vi "PolarizationSimulation.vi"() -> ()   [LabVIEW 2018]
uses:
  <vilib>/Utility/xml.llb/Read From XML File(string).vi
  <vilib>/Utility/xml.llb/Write to XML File(string).vi
  <vilib>/Analysis/NI_AALBase.lvlib
panel:
  out "NN Testing Error":dbl(graph)
  in  "Optimizer":enum16{"Adagrad", "Adadelta", "Adam"}(ring)
  in  "Loss Function":enum16{"MSE", "MAE"}(ring)
  in  "Parameters File Path":path
  out "NN Error":dbl
  in  "Training?":bool
  out "NN Output":dbl
  in  "Speed\nMultiplier":dbl=1.0
  out "Rho_-":cluster{dbl[], "Array 3":dbl[]}(graph)
  out "Rho_0":cluster{dbl[], "Array out":dbl[]}(graph)
  in  "AFP On":bool
  in  "AFP Efficiency":dbl=0.9 min=0.0 max=1.0 step=0.01
  in  "AFP Control":cluster{i32, i32}(slide)={200, 230} scale=0.0..500.0
  out "lower R-value AFP":dbl
  out "upper R-value AFP":dbl
  in  "STOP":bool
  in  "Microwave Power":dbl=1.0
  in  "Lower Fit\nParameter":dbl=-3.6
  in  "Upper Fit\nParameter":dbl=3.6
  in  "Std Dev Noise":dbl step=0.0001
  out "lower R-value":dbl
  out "upper R-value":dbl
  in  "RF Control":cluster{i32, i32}(slide)={200, 230} scale=0.0..500.0
  out "p":dbl format="%_4g"
  out "r":dbl
  in  "Saturation\nPolarization":dbl=0.8 min=0.0 max=0.99 step=0.01
  out "Reimann \nsum of Q":dbl format="%_4g"
  out "Corrected Data (Q)":cluster{dbl[], dbl[]}(graph)
  out "Rho_+":cluster{dbl[], "Array out":dbl[]}(graph)
  in  "Select Target Type":u16(ring)=2 items=["Test Case", "Deuteron"]
  in  "Reset":bool
  out "Total Polarization (P)":cluster{dbl, dbl}(graph)
  in  "Spin Manipulation\nPower Factor":dbl=0.005
  in  "Decay Spin\nManipulation":bool
  out "Reimann\nsum of P":dbl format="%_4g"
  out "Corrected Data (P)":cluster{dbl[], dbl[]}[](graph)
  out "Signal and Fit (P)":cluster{dbl[], "Best Polynomial Fit":dbl[]}[](graph)
  in  "Positive\nPolarization":bool
  in  "Microwave on":bool
  # "Neural Network"
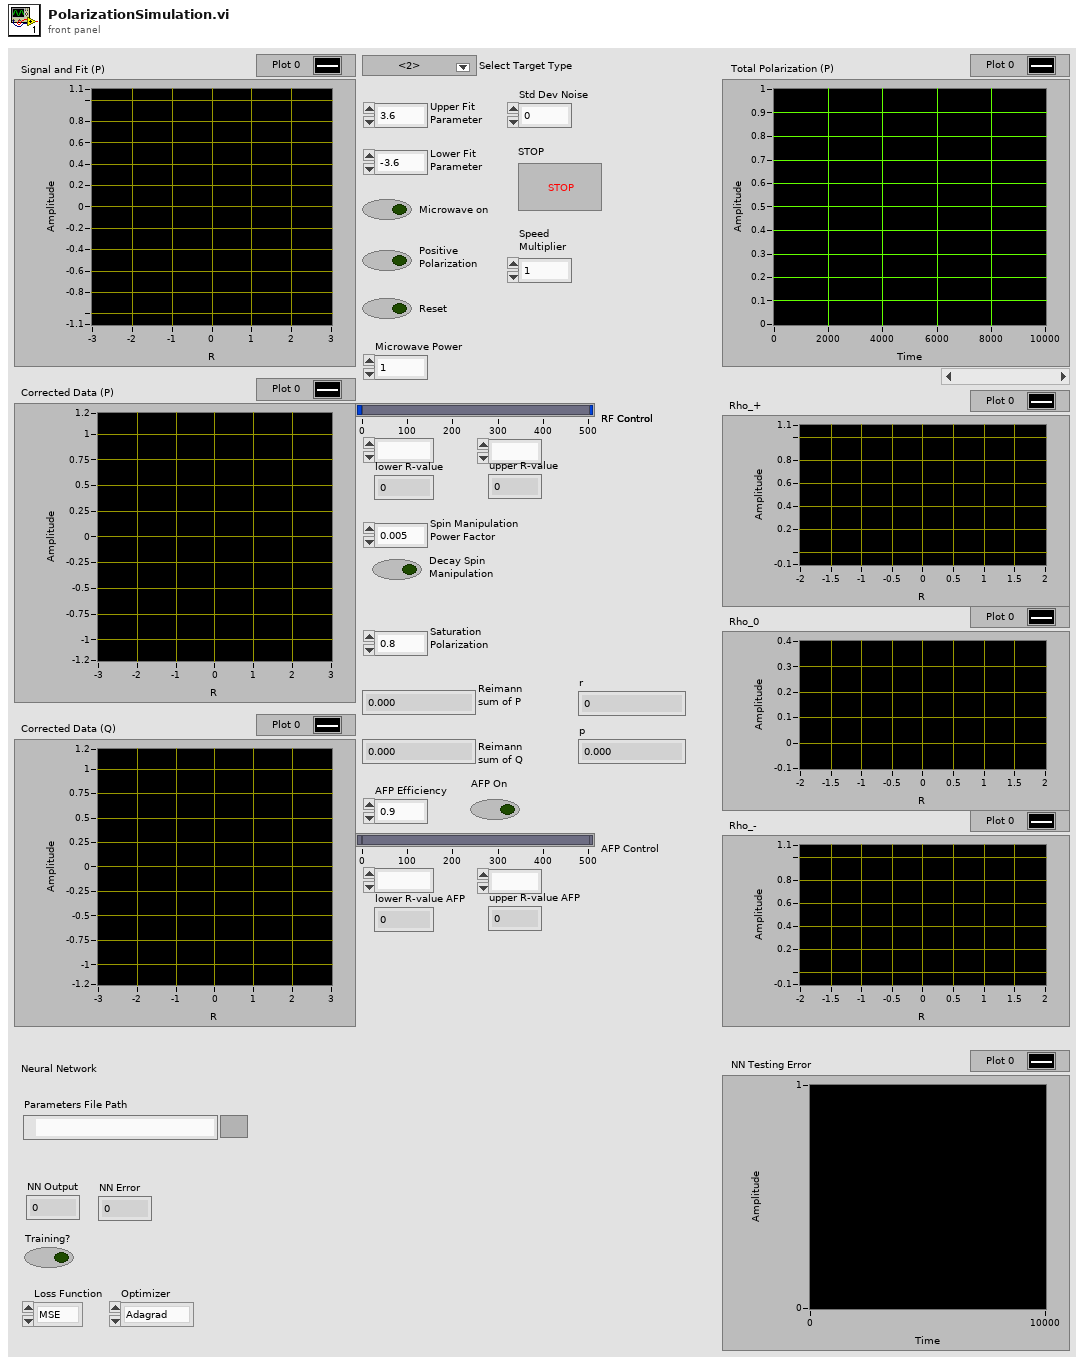
[diagram p1: front panel]
types:
  T1 = cluster{"Mw Moments":cluster{"3 ":dbl[], "2":dbl[][], "1":dbl[][]}, "Vw Moments":cluster{"3":dbl[], "2":dbl[][], "1":dbl[][]}, "Mb Moments":cluster{"1":dbl[], "2":dbl[], "3":dbl}, "Vb Moments":cluster{"3":dbl, "2":dbl[], "1":dbl[]}}
  T2 = cluster{cluster{dbl[][], dbl[]}, cluster{dbl[][], dbl[]}, cluster{dbl[], dbl}}
  T3 = cluster{cluster{"Updated Weights":dbl[][], "Updated Biases":dbl[]}, cluster{"Updated Weights":dbl[][], "Updated Biases":dbl[]}, cluster{"Updated Weights":dbl[], "Updated Biases":dbl}}
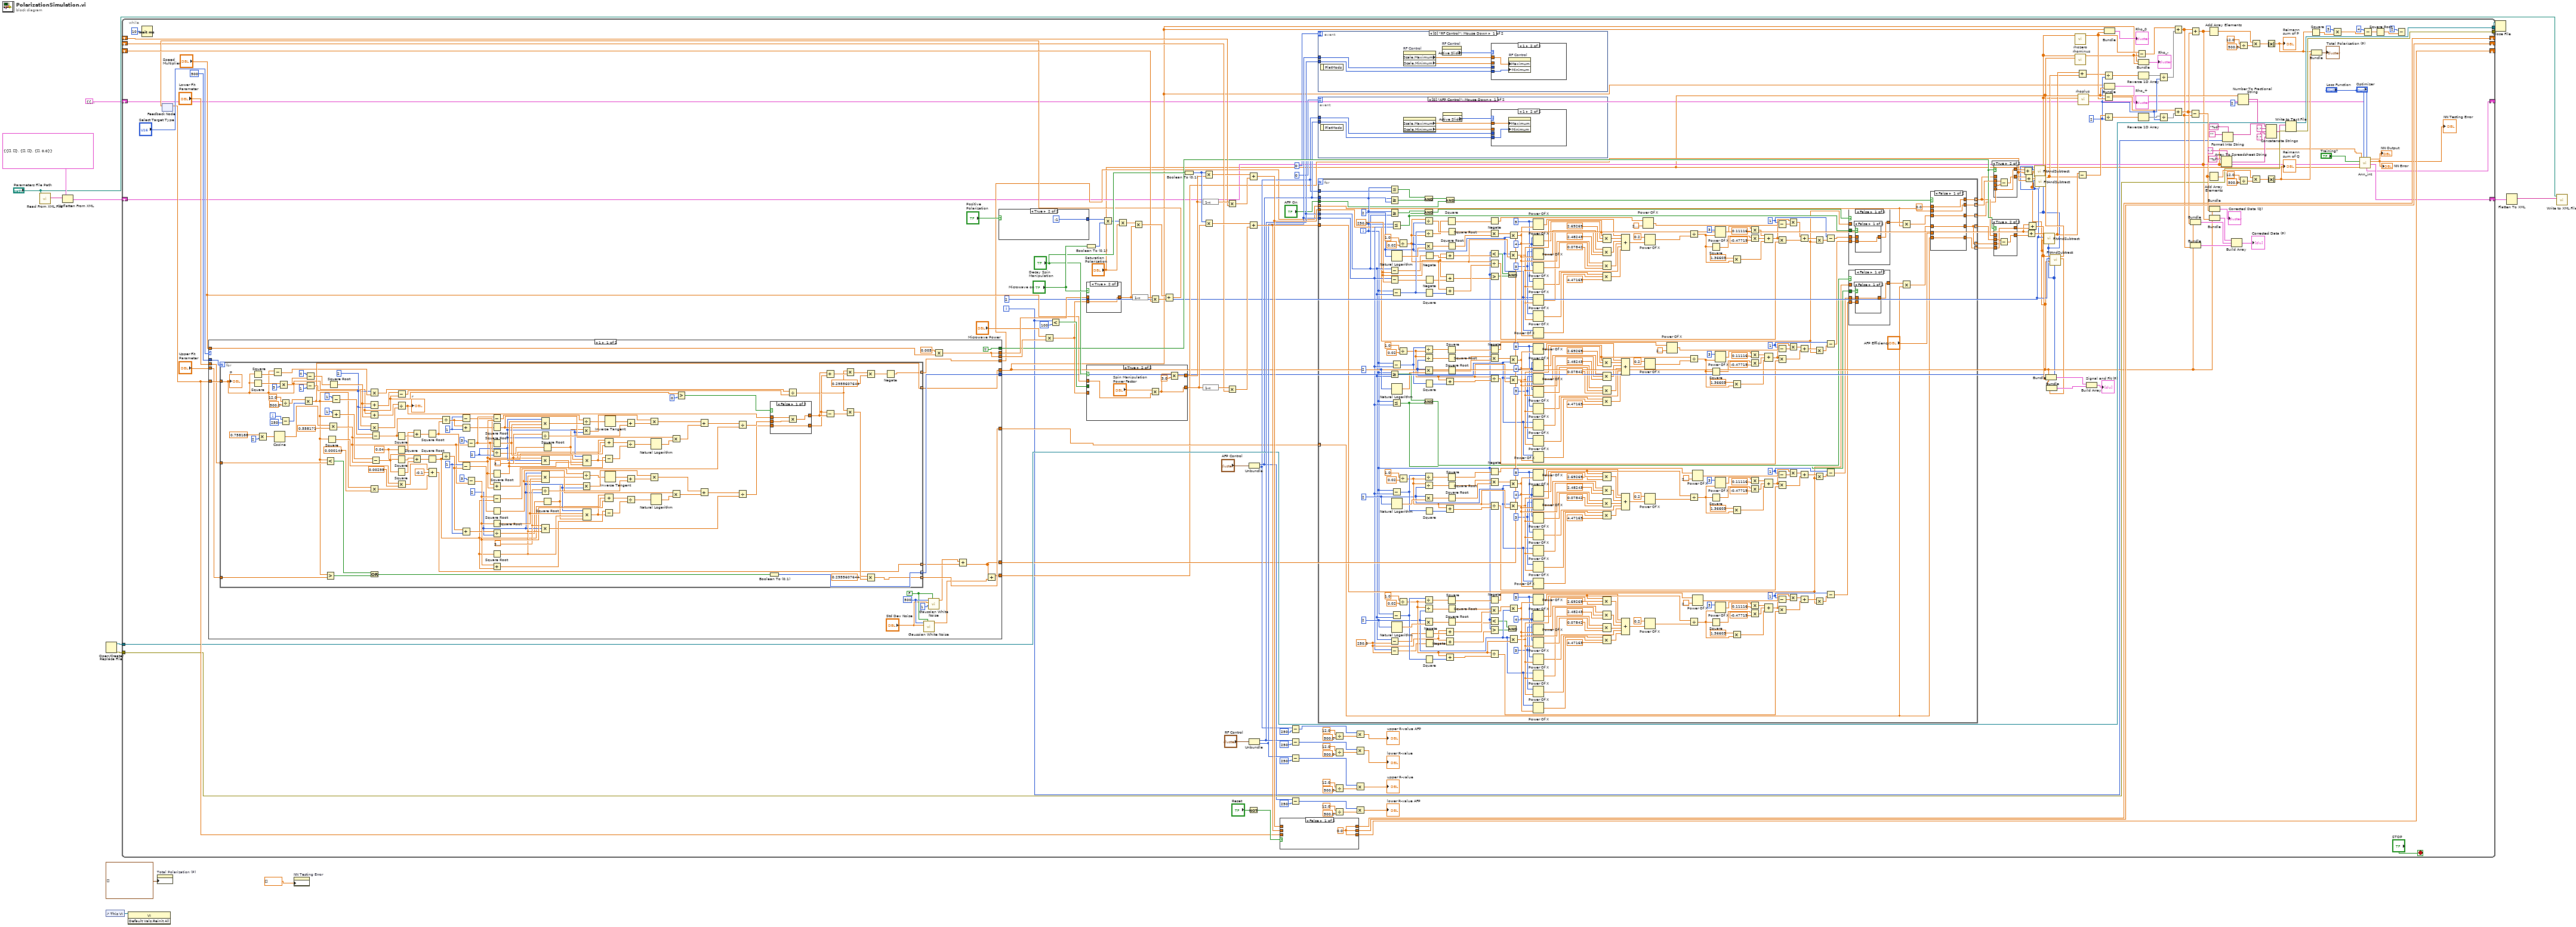
[diagram p0: block diagram]
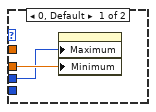
[diagram p2: hidden frame]
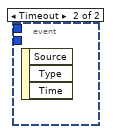
[diagram p3: hidden frame]
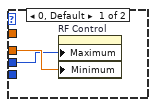
[diagram p4: hidden frame]
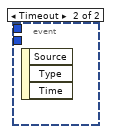
[diagram p5: hidden frame]
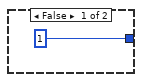
[diagram p6: hidden frame]
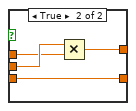
[diagram p7: hidden frame]
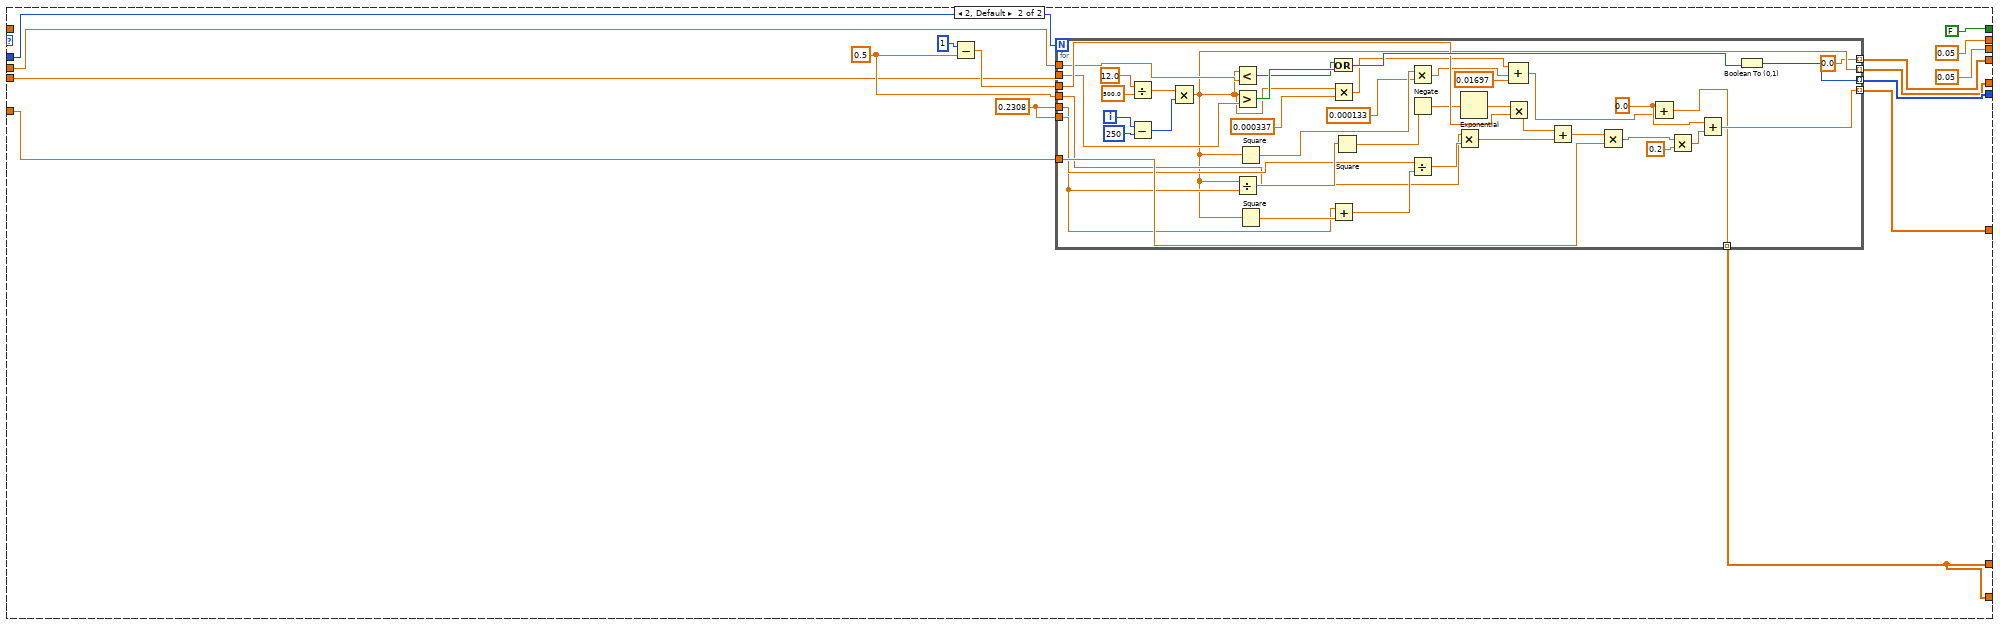
[diagram p8: hidden frame]
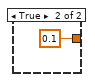
[diagram p10: hidden frame]
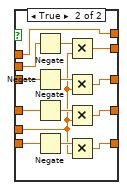
[diagram p15: hidden frame]
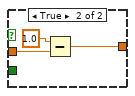
[diagram p17: hidden frame]
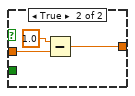
[diagram p19: hidden frame]
diagram:
  n1 = call-poly <vilib>:"Read From XML File.vi"("XML File Path"="Parameters File Path") -> ("XML Elements"=w8:string)  [unwired: 8 in, 2 out]
  n2 = Unflatten From XML(xml string=w8, type=T2 {{[], []}, {[], []}, {[], 0.0}}) -> (value=w6:T2)  [unwired: 1 in, 1 out]
  n3 = Open/Create/Replace File() -> (refnum out=w12:refnum<file>, error out=w11:errorcluster)  [unwired: 6 in, 1 out]
  n4 = control-ref of="This VI"() -> (w14:refnum<vi>)
  n5 = while {
    shift-right: [w181] -> _
    shift-left: _ -> [w188]
    shift-right: [w180] -> _
    shift-left: _ -> [w163]
    shift-right: [w158] -> _
    shift-left: _ -> [w157]
    tunnel: w12 -> [w90]
    tunnel: w11 -> [w89]
    tunnel: [w88] -> w10
    tunnel: [w87] -> w9
    shift-right: [w25] -> w5
    shift-left: w6 -> [w24]
    shift-right: [w17] -> _
    shift-left: T1 {"Mw Moments"={"3 "=[], "2"=[], "1"=[]}, "Vw Moments"={"3"=[], "2"=[], "1"=[]}, "Mb Moments"={"1"=[], "2"=[], "3"=0.0}, "Vb Moments"={"3"=0.0, "2"=[], "1"=[]}} -> [w18]
    i -> [w16]
    stop <- "STOP" stop-if-true
    w140 = 2
    w33 = 2
    n6 = Wait (ms)(milliseconds to wait=10) -> ()  [unwired: 1 out]
    n7 = feedback #1() -> (w167:dbl)  [unwired: 1 in]
    n8 = case shown="1" "Select Target Type" {
      tunnel: [w223 0.05 ("Growth Constant")] -> w172
      tunnel: [w223 0.05 ("Decay Constant")] -> w171
      tunnel: 500 -> [w232 w390]
      tunnel: w167 -> [w235 w389]
      tunnel: "Upper Fit\nParameter" -> [w233 w387]
      tunnel: "Lower Fit\nParameter" -> [w234 w388]
      tunnel: [w230 w385] -> w32
      tunnel: [w220 w384] -> w47
      tunnel: [w231 w386] -> w31
      tunnel: [TRUE FALSE] -> w151
      tunnel: [w221 w380] -> w46
      tunnel: "Speed\nMultiplier" -> [w222 _]
      tunnel: [w216 w379] -> w45
      tunnel: [w218 w379] -> w44
      frame 1 {
        w225 = FALSE
        w227 = 500
        n9 = for {
          N: w232 -> [_]
          tunnel: [w266] -> w230 mode=indexing
          tunnel: [w355] -> w231 mode=indexing
          tunnel: w233 -> [w354]
          tunnel: w234 -> [w353]
          tunnel: [w238] -> w220 mode=indexing
          tunnel: w235 -> [w239]
          tunnel: [w237] -> w221 mode=indexing
          tunnel: [w236] -> w219 mode=indexing
          i -> [w331]
          w253 = 2
          w292 = 1
          w296 = 3.141592653589793
          w290 = 2
          w275 = 0.04
          w328 = 1
          w333 = 3.141592653589793
          w326 = 2
          n10 = Square(x=w239) -> (x^2=w256:dbl)
          n11 = Square(x=w239) -> (x^2=w282:dbl)
          n12 = Multiply(x=0.758188, y=2) -> (x*y=w270:dbl)
          n13 = Subtract(x=w239, y=w256) -> (x-y=w255:dbl)
          n14 = Cosine(x=w270) -> (cos(x)=w273:dbl)
          n15 = Multiply(x=w282, y=3) -> (x*y=w281:dbl)
          n16 = Divide(x=12.0, y=500.0) -> (x/y=w369:dbl)
          n17 = Subtract(x=w331, y=250) -> (x-y=w368:i32)
          n18 = Multiply(x=w369, y=w368) -> (x*y=w266:dbl)
          n19 = Subtract(x=4, y=w281) -> (x-y=w279:dbl)
          n20 = Subtract(x=w239, y=1) -> (x-y=w277:dbl)
          n21 = Less?(x=w266, y=w353) -> (x < y?=w358:bool)
          n22 = Greater?(x=w266, y=w354) -> (0:w357:bool)
          n23 = Square(x=w266) -> (x^2=w268:dbl)
          n24 = Multiply(x=w273, y=0.558171) -> (x*y=w274:dbl)
          n25 = Square Root(x=w279) -> (sqrt(x)=w254:dbl)
          n26 = Subtract(x=1, y=w266) -> (x-y=w363:dbl)
          n27 = Add(x=1, y=w266) -> (x+y=w320:dbl)
          n28 = Multiply(x=w253, y=w255) -> (x*y=w251:dbl)
          n29 = Add(x=w254, y=w253) -> (x+y=w252:dbl)
          n30 = Add(x=w239, y=w254) -> (x+y=w278:dbl)
          n31 = Multiply(x=w277, y=w253) -> (x*y=w261:dbl)
          n32 = Multiply(x=w266, y=0.000144) -> (x*y=w263:dbl)
          n33 = Or(x=w358, y=w357) -> (x .or. y?=w356:bool)
          n34 = Subtract(x=w363, y=w274) -> (x-y=w359:dbl)
          n35 = Subtract(x=w320, y=w274) -> (x-y=w316:dbl)
          n36 = Square(x=w359) -> (x^2=w362:dbl)
          n37 = Square(x=w275) -> (x^2=w361:dbl)
          n38 = Square(x=w275) -> (x^2=w318:dbl)
          n39 = Square(x=w316) -> (x^2=w319:dbl)
          n40 = Subtract(x=w252, y=w239) -> (x-y=w250:dbl)
          n41 = Divide(x=w278, y=w261) -> (x/y=w257:dbl)
          "r" <- w257
          n42 = Multiply(x=w268, y=0.00295) -> (x*y=w267:dbl)
          n43 = Add(x=w361, y=w362) -> (x+y=w360:dbl)
          n44 = Add(x=w318, y=w319) -> (x+y=w317:dbl)
          n45 = Square Root(x=w360) -> (sqrt(x)=w323:dbl)
          n46 = Square Root(x=w317) -> (sqrt(x)=w287:dbl)
          n47 = Compound Arithmetic op=ADD(w267, -0.1, w263) -> (w236:dbl)
          n48 = Divide(x=w359, y=w323) -> (x/y=w329:dbl)
          n49 = Divide(x=w316, y=w287) -> (x/y=w293:dbl)
          n50 = Subtract(x=w328, y=w329) -> (x-y=w284:dbl)
          n51 = Add(x=w329, y=w328) -> (x+y=w327:dbl)
          n52 = Subtract(x=w292, y=w293) -> (x-y=w285:dbl)
          n53 = Add(x=w293, y=w292) -> (x+y=w291:dbl)
          n54 = Subtract(x=3, y=w274) -> (x-y=w339:dbl)
          n55 = Subtract(x=3, y=w274) -> (x-y=w302:dbl)
          n56 = Subtract(x=w339, y=w323) -> (x-y=w348:dbl)
          n57 = Square Root(x=w284) -> (sqrt(x)=w330:dbl)
          n58 = Square Root(x=w339) -> (sqrt(x)=w342:dbl)
          n59 = Divide(x=w327, y=w326) -> (x/y=w325:dbl)
          n60 = Square Root(x=w323) -> (sqrt(x)=w332:dbl)
          n61 = Add(x=w339, y=w323) -> (x+y=w338:dbl)
          n62 = Subtract(x=w302, y=w287) -> (x-y=w311:dbl)
          n63 = Square Root(x=w285) -> (sqrt(x)=w294:dbl)
          n64 = Square Root(x=w302) -> (sqrt(x)=w305:dbl)
          n65 = Divide(x=w291, y=w290) -> (x/y=w289:dbl)
          n66 = Square Root(x=w287) -> (sqrt(x)=w295:dbl)
          n67 = Add(x=w302, y=w287) -> (x+y=w301:dbl)
          n68 = Divide(x=w333, y=w326) -> (x/y=w350:dbl)
          n69 = Divide(x=w296, y=w290) -> (x/y=w313:dbl)
          n70 = Compound Arithmetic op=MULTIPLY(w326, w332, w342, w330) -> (w347:dbl)
          n71 = Compound Arithmetic op=MULTIPLY(w333, w326, w332) -> (w334:dbl)
          n72 = Compound Arithmetic op=MULTIPLY(w290, w295, w305, w294) -> (w310:dbl)
          n73 = Compound Arithmetic op=MULTIPLY(w296, w290, w295) -> (w297:dbl)
          n74 = Square Root(x=w325) -> (sqrt(x)=w324:dbl)
          n75 = Square Root(x=w289) -> (sqrt(x)=w288:dbl)
          n76 = Divide(x=w348, y=w347) -> (x/y=w346:dbl)
          n77 = Multiply(x=w324, y=w326) -> (x*y=w352:dbl)
          n78 = Divide(x=w311, y=w310) -> (x/y=w309:dbl)
          n79 = Multiply(x=w288, y=w290) -> (x*y=w315:dbl)
          n80 = Compound Arithmetic op=MULTIPLY(w326, w342, w332, w324) -> (w337:dbl)
          n81 = Compound Arithmetic op=MULTIPLY(w290, w305, w295, w288) -> (w300:dbl)
          n82 = Subtract(x=w338, y=w337) -> (x-y=w336:dbl)
          n83 = Subtract(x=w301, y=w300) -> (x-y=w299:dbl)
          n84 = Inverse Tangent(1:w346) -> (0:w351:dbl)
          n85 = Compound Arithmetic op=ADD(w337, w323, w339) -> (w341:dbl)
          n86 = Inverse Tangent(1:w309) -> (0:w314:dbl)
          n87 = Compound Arithmetic op=ADD(w300, w287, w302) -> (w304:dbl)
          n88 = Add(x=w351, y=w350) -> (x+y=w349:dbl)
          n89 = Divide(x=w341, y=w336) -> (x/y=w340:dbl)
          n90 = Add(x=w314, y=w313) -> (x+y=w312:dbl)
          n91 = Divide(x=w304, y=w299) -> (x/y=w303:dbl)
          n92 = Multiply(x=w352, y=w349) -> (x*y=w345:dbl)
          n93 = Multiply(x=w315, y=w312) -> (x*y=w308:dbl)
          n94 = Natural Logarithm(1:w340) -> (0:w343:dbl)
          n95 = Natural Logarithm(1:w303) -> (0:w306:dbl)
          n96 = Multiply(x=w330, y=w343) -> (x*y=w344:dbl)
          n97 = Multiply(x=w294, y=w306) -> (x*y=w307:dbl)
          n98 = Greater?(x=w239, y=0) -> (0:w241:bool)
          n99 = Add(x=w345, y=w344) -> (x+y=w335:dbl)
          n100 = Add(x=w308, y=w307) -> (x+y=w298:dbl)
          n101 = Divide(x=w335, y=w334) -> (x/y=w276:dbl)
          n102 = Divide(x=w298, y=w297) -> (x/y=w243:dbl)
          n103 = Boolean To (0,1)(Boolean=w356) -> (0, 1=w355:i16)
          n104 = case shown="False" w241 {
            tunnel: w276 -> [w373 w378]
            tunnel: [w371 w377] -> w259
            tunnel: w257 -> [w374 w376]
            tunnel: w243 -> [w372 w375]
            tunnel: [w372 w375] -> w242
            frame False {
              n105 = Multiply(x=w374, y=w373) -> (x*y=w371:dbl)
            }
            frame True {
              n106 = Multiply(x=w378, y=w376) -> (x*y=w377:dbl)
            }
          }
          n107 = Divide(x=w251, y=w250) -> (x/y=w249:dbl)
          n108 = Add(x=w259, y=w242) -> (x+y=w260:dbl)
          n109 = Subtract(x=w242, y=w259) -> (x-y=w286:dbl)
          n110 = Multiply(x=w249, y=w260) -> (x*y=w248:dbl)
          n111 = Multiply(x=w249, y=w286) -> (x*y=w247:dbl)
          n112 = Multiply(x=w248, y=0.2955607644) -> (x*y=w246:dbl)
          n113 = Multiply(x=w247, y=0.2955607644) -> (x*y=w238:dbl)
          n114 = Negate(x=w246) -> (-x=w237:dbl)
          "p" <- w239
        }
        n115 = call <vilib>:"Gaussian White Noise.vi"("initialize?"=w225, "standard deviation"="Std Dev Noise", "samples"=w227) -> ("Gaussian noise pattern"=w217:dbl[])  [unwired: 7 in, 1 out]
        n116 = call <vilib>:"Gaussian White Noise.vi"("initialize?"=w225, "seed"=1, "standard deviation"="Std Dev Noise", "samples"=w227) -> ("Gaussian noise pattern"=w215:dbl[])  [unwired: 6 in, 1 out]
        n117 = Multiply(x=0.005, y=w222) -> (x*y=w223:dbl)
        n118 = Add(x=w215, y=w219) -> (x+y=w216:dbl[])
        n119 = Add(x=w216, y=w217) -> (x+y=w218:dbl[])
      }
      frame 2, Default {
        w391 = 0.2308
        w392 = 0.5
        n120 = Subtract(x=1, y=w392) -> (x-y=w394:dbl)
        n121 = for {
          N: w390 -> [_]
          tunnel: w389 -> [w434]
          tunnel: [w400] -> w385 mode=indexing
          tunnel: [w418] -> w384 mode=indexing
          tunnel: [w432] -> w386 mode=indexing
          tunnel: w394 -> [w428]
          tunnel: w391 -> [w426]
          tunnel: w391 -> [w407]
          tunnel: w392 -> [w420]
          tunnel: w387 -> [w415]
          tunnel: w388 -> [w414]
          tunnel: [0.0] -> w380 mode=indexing
          tunnel: [w395] -> w379 mode=indexing
          i -> [w408]
          w419 = 0.0
          n122 = Divide(x=12.0, y=500.0) -> (x/y=w409:dbl)
          n123 = Subtract(x=w408, y=250) -> (x-y=w413:i32)
          n124 = Multiply(x=w409, y=w413) -> (x*y=w400:dbl)
          n125 = Less?(x=w400, y=w414) -> (x < y?=w429:bool)
          n126 = Greater?(x=w400, y=w415) -> (0:w430:bool)
          n127 = Divide(x=w400, y=w407) -> (x/y=w435:dbl)
          n128 = Square(x=w400) -> (x^2=w403:dbl)
          n129 = Square(x=w400) -> (x^2=w425:dbl)
          n130 = Or(x=w429, y=w430) -> (x .or. y?=w431:bool)
          n131 = Multiply(x=w400, y=0.000337) -> (x*y=w402:dbl)
          n132 = Add(x=w407, y=w425) -> (x+y=w427:dbl)
          n133 = Square(x=w435) -> (x^2=w436:dbl)
          n134 = Multiply(x=w403, y=0.000133) -> (x*y=w401:dbl)
          n135 = Negate(x=w436) -> (-x=w417:dbl)
          n136 = Divide(x=w426, y=w427) -> (x/y=w422:dbl)
          n137 = Multiply(x=w420, y=w422) -> (x*y=w421:dbl)
          n138 = Exponential(1:w417) -> (0:w416:dbl)
          n139 = Multiply(x=w416, y=w428) -> (x*y=w424:dbl)
          n140 = Compound Arithmetic op=ADD(w402, w401, 0.01697) -> (w404:dbl)
          n141 = Add(x=w424, y=w421) -> (x+y=w423:dbl)
          n142 = Multiply(x=w423, y=w434) -> (x*y=w433:dbl)
          n143 = Add(x=w419, y=w404) -> (x+y=w395:dbl)
          n144 = Multiply(x=w433, y=0.2) -> (x*y=w406:dbl)
          n145 = Add(x=w419, y=w406) -> (x+y=w418:dbl)
          n146 = Boolean To (0,1)(Boolean=w431) -> (0, 1=w432:i16)
        }
      }
    }
    n147 = case shown="True" "Positive\nPolarization" {
      tunnel: [1 -1] -> w125
      frame False {
      }
      frame True {
      }
    }
    n148 = Multiply(x="Microwave Power", y=w172) -> (x*y=w93:dbl)
    n149 = Less?(x=w16, y=100) -> (x < y?=w183:bool)
    n150 = Boolean To (0,1)(Boolean="Microwave on") -> (0, 1=w190:i16)
    n151 = case shown="True" "Microwave on" {
      tunnel: [w447 w448] -> w175
      tunnel: w93 -> [_ w448]
      tunnel: w171 -> [w447 _]
      frame False {
      }
      frame True {
      }
    }
    n152 = case shown="True" "Decay Spin\nManipulation" {
      tunnel: [w437 w443] -> w184
      tunnel: w93 -> [w439 _]
      tunnel: w183 -> [w438 _]
      tunnel: [w437 w444] -> w165
      tunnel: "Speed\nMultiplier" -> [_ w442]
      frame False {
        n153 = case shown="False" w438 {
          tunnel: [w440 0.1] -> w437
          tunnel: w439 -> [w440 _]
          frame False {
          }
          frame True {
          }
        }
      }
      frame True {
        n154 = Multiply(x="Spin Manipulation\nPower Factor", y=w442) -> (x*y=w443:dbl)
        n155 = Multiply(x=w443, y=3.0) -> (x*y=w444:dbl)
      }
    }
    n156 = Multiply(x=w125, y=w190) -> (x*y=w126:i32)
    n157 = Multiply(x=w126, y="Saturation\nPolarization") -> (x*y=w133:dbl)
    n158 = expression code="1-x"(w175) -> (w191:dbl)
    n159 = Multiply(x=w133, y=w175) -> (x*y=w192:dbl)
    n160 = Multiply(x=w191, y=w188) -> (x*y=w193:dbl)
    n161 = Add(x=w192, y=w193) -> (x+y=w170:dbl)
    n162 = feedback-in #1(w170) -> ()
    n163 = Boolean To (0,1)(Boolean="Decay Spin\nManipulation") -> (0, 1=w166:i16)
    n164 = expression code="1-x"(w165) -> (w164:dbl)
    n165 = expression code="1-x"(w184) -> (w185:dbl)
    n166 = Multiply(x=w166, y=w165) -> (x*y=w161:dbl)
    n167 = Multiply(x=w166, y=w184) -> (x*y=w186:dbl)
    n168 = Multiply(x=w164, y=w157) -> (x*y=w162:dbl)
    n169 = Multiply(x=w185, y=w163) -> (x*y=w187:dbl)
    n170 = Add(x=w161, y=w162) -> (x+y=w159:dbl)
    n171 = Add(x=w186, y=w187) -> (x+y=w179:dbl)
    n172 = Not(x="Reset") -> (.not. x?=w178:bool)
    n173 = Unbundle("AFP Control") -> (w57:i32, w56:i32)
    n174 = Unbundle("RF Control") -> (w96:i32, w95:i32)
    n175 = case shown="False" w178 {
      tunnel: [w461 w464] -> w181
      tunnel: w167 -> [_ w464]
      tunnel: [w461 w463] -> w180
      tunnel: w179 -> [_ w463]
      tunnel: w159 -> [_ w462]
      tunnel: [w461 w462] -> w158
      frame False {
        w461 = 0.0
      }
      frame True {
      }
    }
    n176 = Subtract(x=w56, y=250) -> (x-y=w63:i32)
    n177 = Subtract(x=w96, y=250) -> (x-y=w102:i32)
    n178 = Subtract(x=w95, y=250) -> (x-y=w105:i32)
    n179 = Subtract(x=w57, y=250) -> (x-y=w60:i32)
    n180 = event shown="[0] \"RF Control\": Mouse Down" {
      selector: _ -> [_ _]
      dyn-events: _ -> [_ _]
      timeout: 0 -> [_ _]
      tunnel: w96 -> [w205 _]
      tunnel: w95 -> [w204 _]
      event "RF Control": Mouse Down {
        n181 = event-data() -> ()  [unwired: 1 in, 1 out]
        n182 = property on="RF Control" class="Slide (strict)"() -> ("Scale.Maximum"=w206:dbl, "Scale.Minimum"=w207:dbl)  [unwired: 2 in, 2 out]
        n183 = property on="RF Control" class="Slide (strict)"() -> ("Active Slider"=w208:i32)  [unwired: 2 in, 2 out]
        n184 = case shown="1" w208 {
          tunnel: w207 -> [w210 _]
          tunnel: w204 -> [w209 _]
          tunnel: w206 -> [_ w212]
          tunnel: w205 -> [_ w211]
          frame 0, Default {
            n185 = property on="RF Control" class="Slide (strict)"("Maximum"=w209, "Minimum"=w210) -> ()  [unwired: 2 in, 2 out]
          }
          frame 1 {
            n186 = property on="RF Control" class="Slide (strict)"("Maximum"=w212, "Minimum"=w211) -> ()  [unwired: 2 in, 2 out]
          }
        }
      }
      event Timeout {
        n187 = event-data() -> ()  [unwired: 1 in, 3 out]
      }
    }
    n188 = event shown="[0] \"AFP Control\": Mouse Down" {
      selector: _ -> [_ _]
      dyn-events: _ -> [_ _]
      timeout: 0 -> [_ _]
      tunnel: w57 -> [w196 _]
      tunnel: w56 -> [w195 _]
      event "AFP Control": Mouse Down {
        n189 = event-data() -> ()  [unwired: 1 in, 1 out]
        n190 = property on="AFP Control" class="Slide (strict)"() -> ("Scale.Maximum"=w197:dbl, "Scale.Minimum"=w198:dbl)  [unwired: 2 in, 2 out]
        n191 = property on="AFP Control" class="Slide (strict)"() -> ("Active Slider"=w199:i32)  [unwired: 2 in, 2 out]
        n192 = case shown="1" w199 {
          tunnel: w198 -> [w201 _]
          tunnel: w195 -> [w200 _]
          tunnel: w197 -> [_ w203]
          tunnel: w196 -> [_ w202]
          frame 0, Default {
            n193 = property on="AFP Control" class="Slide (strict)"("Maximum"=w200, "Minimum"=w201) -> ()  [unwired: 2 in, 2 out]
          }
          frame 1 {
            n194 = property on="AFP Control" class="Slide (strict)"("Maximum"=w203, "Minimum"=w202) -> ()  [unwired: 2 in, 2 out]
          }
        }
      }
      event Timeout {
        n195 = event-data() -> ()  [unwired: 1 in, 3 out]
      }
    }
    n196 = for {
      tunnel: w47 -> [w477] mode=indexing
      tunnel: w179 -> [w629]
      tunnel: w95 -> [w487]
      tunnel: w96 -> [w486]
      tunnel: [w473] -> w169 mode=indexing
      tunnel: [w474] -> w160 mode=indexing
      tunnel: [w474] -> w168 mode=indexing
      tunnel: w46 -> [w466] mode=indexing
      tunnel: w159 -> [w485]
      tunnel: [w465] -> w155 mode=indexing
      tunnel: [w472] -> w145 mode=indexing
      tunnel: w57 -> [w481]
      tunnel: w56 -> [w480]
      tunnel: "AFP On" -> [w469]
      tunnel: [w468] -> w54 mode=indexing
      i -> [w479]
      w489 = 250.0
      w528 = 5
      w526 = 4
      w525 = 3
      w506 = 1
      w507 = 2
      w589 = 5
      w587 = 4
      w586 = 3
      w566 = 1
      w567 = 2
      w623 = 250.0
      w664 = 5
      w662 = 4
      w661 = 3
      w642 = 1
      w643 = 2
      w725 = 5
      w723 = 4
      w722 = 3
      w702 = 1
      w703 = 2
      n197 = Less Or Equal?(x=w479, y=w480) -> (x <= y?=w482:bool)
      n198 = Greater Or Equal?(x=w479, y=w481) -> (x >= y?=w483:bool)
      n199 = Greater Or Equal?(x=w479, y=w486) -> (x >= y?=w562:bool)
      n200 = Subtract(x=w486, y=w489) -> (x-y=w493:dbl)
      n201 = Subtract(x=w487, y=w489) -> (x-y=w494:dbl)
      n202 = Greater Or Equal?(x=w479, y=w486) -> (x >= y?=w698:bool)
      n203 = Subtract(x=w486, y=w623) -> (x-y=w627:dbl)
      n204 = Subtract(x=w487, y=w623) -> (x-y=w628:dbl)
      n205 = Less Or Equal?(x=w479, y=w487) -> (x <= y?=w499:bool)
      n206 = Natural Logarithm(1:w567) -> (0:w602:dbl)
      n207 = Subtract(x=w479, y=w486) -> (x-y=w575:i32)
      n208 = Subtract(x=w479, y=w487) -> (x-y=w514:i32)
      n209 = Natural Logarithm(1:w507) -> (0:w541:dbl)
      n210 = Less Or Equal?(x=w479, y=w487) -> (x <= y?=w634:bool)
      n211 = Subtract(x=w479, y=w487) -> (x-y=w650:i32)
      n212 = Natural Logarithm(1:w643) -> (0:w677:dbl)
      n213 = Subtract(x=w479, y=w486) -> (x-y=w711:i32)
      n214 = Natural Logarithm(1:w703) -> (0:w738:dbl)
      n215 = Divide(x=1.0, y=0.02) -> (x/y=w571:dbl)
      n216 = Divide(x=1.0, y=0.02) -> (x/y=w511:dbl)
      n217 = Divide(x=1.0, y=0.02) -> (x/y=w647:dbl)
      n218 = Divide(x=1.0, y=0.02) -> (x/y=w707:dbl)
      n219 = And(x=w482, y=w483) -> (x .and. y?=w471:bool)
      n220 = And(x=w562, y=w499) -> (x .and. y?=w500:bool)
      n221 = Divide(x=w571, y=w567) -> (x/y=w600:dbl)
      n222 = Divide(x=w575, y=w571) -> (x/y=w579:dbl)
      n223 = Multiply(x=w567, y=w602) -> (x*y=w603:dbl)
      n224 = Divide(x=w514, y=w511) -> (x/y=w518:dbl)
      n225 = Divide(x=w511, y=w507) -> (x/y=w539:dbl)
      n226 = Multiply(x=w507, y=w541) -> (x*y=w542:dbl)
      n227 = And(x=w698, y=w634) -> (x .and. y?=w636:bool)
      n228 = Divide(x=w650, y=w647) -> (x/y=w654:dbl)
      n229 = Divide(x=w647, y=w643) -> (x/y=w675:dbl)
      n230 = Multiply(x=w643, y=w677) -> (x*y=w678:dbl)
      n231 = Divide(x=w711, y=w707) -> (x/y=w715:dbl)
      n232 = Divide(x=w707, y=w703) -> (x/y=w736:dbl)
      n233 = Multiply(x=w703, y=w738) -> (x*y=w739:dbl)
      n234 = Square(x=w575) -> (x^2=w576:i32)
      n235 = Square(x=w514) -> (x^2=w515:i32)
      n236 = Square(x=w650) -> (x^2=w651:i32)
      n237 = Square(x=w711) -> (x^2=w712:i32)
      n238 = Negate(x=w493) -> (-x=w492:dbl)
      n239 = Negate(x=w494) -> (-x=w490:dbl)
      n240 = Negate(x=w627) -> (-x=w626:dbl)
      n241 = Negate(x=w628) -> (-x=w624:dbl)
      n242 = Add(x=w489, y=w492) -> (x+y=w491:dbl)
      n243 = Add(x=w489, y=w490) -> (x+y=w488:dbl)
      n244 = Add(x=w571, y=w576) -> (x+y=w577:dbl)
      n245 = Add(x=w511, y=w515) -> (x+y=w516:dbl)
      n246 = Add(x=w647, y=w651) -> (x+y=w652:dbl)
      n247 = Add(x=w623, y=w626) -> (x+y=w625:dbl)
      n248 = Add(x=w623, y=w624) -> (x+y=w622:dbl)
      n249 = Add(x=w707, y=w712) -> (x+y=w713:dbl)
      n250 = And(x=w471, y=w469) -> (x .and. y?=w470:bool)
      n251 = Square(x=w579) -> (x^2=w581:dbl)
      n252 = Square(x=w518) -> (x^2=w520:dbl)
      n253 = Square(x=w654) -> (x^2=w656:dbl)
      n254 = Square(x=w715) -> (x^2=w717:dbl)
      n255 = Square Root(x=w600) -> (sqrt(x)=w601:dbl)
      n256 = Square Root(x=w603) -> (sqrt(x)=w604:dbl)
      n257 = Square Root(x=w539) -> (sqrt(x)=w540:dbl)
      n258 = Square Root(x=w542) -> (sqrt(x)=w543:dbl)
      n259 = Square Root(x=w675) -> (sqrt(x)=w676:dbl)
      n260 = Square Root(x=w678) -> (sqrt(x)=w679:dbl)
      n261 = Square Root(x=w736) -> (sqrt(x)=w737:dbl)
      n262 = Square Root(x=w739) -> (sqrt(x)=w740:dbl)
      n263 = Negate(x=w581) -> (-x=w580:dbl)
      n264 = Multiply(x=w601, y=w604) -> (x*y=w595:dbl)
      n265 = Less?(x=w479, y=w491) -> (x < y?=w496:bool)
      n266 = Divide(x=w571, y=w577) -> (x/y=w574:dbl)
      n267 = Greater?(x=w479, y=w488) -> (0:w495:bool)
      n268 = Negate(x=w520) -> (-x=w519:dbl)
      n269 = Multiply(x=w540, y=w543) -> (x*y=w534:dbl)
      n270 = Divide(x=w511, y=w516) -> (x/y=w501:dbl)
      n271 = Negate(x=w656) -> (-x=w655:dbl)
      n272 = Multiply(x=w676, y=w679) -> (x*y=w670:dbl)
      n273 = Divide(x=w647, y=w652) -> (x/y=w637:dbl)
      n274 = Negate(x=w717) -> (-x=w716:dbl)
      n275 = Multiply(x=w737, y=w740) -> (x*y=w731:dbl)
      n276 = Less?(x=w479, y=w625) -> (x < y?=w631:bool)
      n277 = Greater?(x=w479, y=w622) -> (0:w630:bool)
      n278 = Divide(x=w707, y=w713) -> (x/y=w710:dbl)
      n279 = And(x=w496, y=w495) -> ()  [unwired: 1 out]
      n280 = And(x=w631, y=w630) -> ()  [unwired: 1 out]
      n281 = Multiply(x=w595, y=w567) -> (x*y=w619:dbl)
      n282 = Multiply(x=w567, y=w571) -> (x*y=w613:dbl)
      n283 = Multiply(x=w534, y=w507) -> (x*y=w558:dbl)
      n284 = Multiply(x=w507, y=w511) -> (x*y=w552:dbl)
      n285 = Multiply(x=w670, y=w643) -> (x*y=w694:dbl)
      n286 = Multiply(x=w643, y=w647) -> (x*y=w688:dbl)
      n287 = Multiply(x=w731, y=w703) -> (x*y=w755:dbl)
      n288 = Multiply(x=w703, y=w707) -> (x*y=w749:dbl)
      n289 = Power Of X(1:w619, 2:w589) -> (0:w606:dbl)
      n290 = Power Of X(1:w619, 2:w587) -> (0:w612:dbl)
      n291 = Power Of X(1:w619, 2:w586) -> (0:w614:dbl)
      n292 = Power Of X(1:w613, 2:w587) -> (0:w618:dbl)
      n293 = Power Of X(1:w613, 2:w589) -> (0:w607:dbl)
      n294 = Power Of X(1:w613, 2:w567) -> (0:w615:dbl)
      n295 = Power Of X(1:w613, 2:w586) -> (0:w616:dbl)
      n296 = Power Of X(1:w619, 2:w567) -> (0:w617:dbl)
      n297 = Power Of X(1:w558, 2:w528) -> (0:w545:dbl)
      n298 = Power Of X(1:w558, 2:w526) -> (0:w551:dbl)
      n299 = Power Of X(1:w558, 2:w525) -> (0:w553:dbl)
      n300 = Power Of X(1:w552, 2:w526) -> (0:w557:dbl)
      n301 = Power Of X(1:w552, 2:w528) -> (0:w546:dbl)
      n302 = Power Of X(1:w552, 2:w507) -> (0:w554:dbl)
      n303 = Power Of X(1:w552, 2:w525) -> (0:w555:dbl)
      n304 = Power Of X(1:w558, 2:w507) -> (0:w556:dbl)
      n305 = Power Of X(1:w694, 2:w664) -> (0:w681:dbl)
      n306 = Power Of X(1:w694, 2:w662) -> (0:w687:dbl)
      n307 = Power Of X(1:w694, 2:w661) -> (0:w689:dbl)
      n308 = Power Of X(1:w688, 2:w662) -> (0:w693:dbl)
      n309 = Power Of X(1:w688, 2:w664) -> (0:w682:dbl)
      n310 = Power Of X(1:w688, 2:w643) -> (0:w690:dbl)
      n311 = Power Of X(1:w688, 2:w661) -> (0:w691:dbl)
      n312 = Power Of X(1:w694, 2:w643) -> (0:w692:dbl)
      n313 = Power Of X(1:w755, 2:w725) -> (0:w742:dbl)
      n314 = Power Of X(1:w755, 2:w723) -> (0:w748:dbl)
      n315 = Power Of X(1:w755, 2:w722) -> (0:w750:dbl)
      n316 = Power Of X(1:w749, 2:w723) -> (0:w754:dbl)
      n317 = Power Of X(1:w749, 2:w725) -> (0:w743:dbl)
      n318 = Power Of X(1:w749, 2:w703) -> (0:w751:dbl)
      n319 = Power Of X(1:w749, 2:w722) -> (0:w752:dbl)
      n320 = Power Of X(1:w755, 2:w703) -> (0:w753:dbl)
      n321 = Compound Arithmetic op=MULTIPLY(w613, w612, 2.69269) -> (w608:dbl)
      n322 = Compound Arithmetic op=MULTIPLY(w614, w615, 2.48243) -> (w610:dbl)
      n323 = Compound Arithmetic op=MULTIPLY(w619, w618, 0.07842) -> (w609:dbl)
      n324 = Compound Arithmetic op=MULTIPLY(w616, w617, 4.47163) -> (w611:dbl)
      n325 = Compound Arithmetic op=MULTIPLY(w552, w551, 2.69269) -> (w547:dbl)
      n326 = Compound Arithmetic op=MULTIPLY(w553, w554, 2.48243) -> (w549:dbl)
      n327 = Compound Arithmetic op=MULTIPLY(w558, w557, 0.07842) -> (w548:dbl)
      n328 = Compound Arithmetic op=MULTIPLY(w555, w556, 4.47163) -> (w550:dbl)
      n329 = Compound Arithmetic op=MULTIPLY(w688, w687, 2.69269) -> (w683:dbl)
      n330 = Compound Arithmetic op=MULTIPLY(w689, w690, 2.48243) -> (w685:dbl)
      n331 = Compound Arithmetic op=MULTIPLY(w694, w693, 0.07842) -> (w684:dbl)
      n332 = Compound Arithmetic op=MULTIPLY(w691, w692, 4.47163) -> (w686:dbl)
      n333 = Compound Arithmetic op=MULTIPLY(w749, w748, 2.69269) -> (w744:dbl)
      n334 = Compound Arithmetic op=MULTIPLY(w750, w751, 2.48243) -> (w746:dbl)
      n335 = Compound Arithmetic op=MULTIPLY(w755, w754, 0.07842) -> (w745:dbl)
      n336 = Compound Arithmetic op=MULTIPLY(w752, w753, 4.47163) -> (w747:dbl)
      n337 = Compound Arithmetic op=unknown(w606, w608, w610, w609, w607, w611) -> (w568:dbl)
      n338 = Compound Arithmetic op=unknown(w545, w547, w549, w548, w546, w550) -> (w508:dbl)
      n339 = Compound Arithmetic op=unknown(w681, w683, w685, w684, w682, w686) -> (w644:dbl)
      n340 = Compound Arithmetic op=unknown(w742, w744, w746, w745, w743, w747) -> (w704:dbl)
      n341 = Power Of X(1:2.718281828459045, 2:w580) -> (0:w578:dbl)
      n342 = Power Of X(1:w568, 2:0.2) -> (0:w621:dbl)
      n343 = Power Of X(1:w508, 2:0.2) -> (0:w560:dbl)
      n344 = Power Of X(1:w644, 2:0.2) -> (0:w696:dbl)
      n345 = Power Of X(1:w704, 2:0.2) -> (0:w757:dbl)
      n346 = Power Of X(1:2.718281828459045, 2:w519) -> (0:w517:dbl)
      n347 = Divide(x=w613, y=w621) -> (x/y=w605:dbl)
      n348 = Divide(x=w552, y=w560) -> (x/y=w544:dbl)
      n349 = Divide(x=w688, y=w696) -> (x/y=w680:dbl)
      n350 = Divide(x=w749, y=w757) -> (x/y=w741:dbl)
      n351 = Power Of X(1:2.718281828459045, 2:w655) -> (0:w653:dbl)
      n352 = Power Of X(1:2.718281828459045, 2:w716) -> (0:w714:dbl)
      n353 = Square(x=w605) -> (x^2=w599:dbl)
      n354 = Square(x=w544) -> (x^2=w538:dbl)
      n355 = Square(x=w680) -> (x^2=w674:dbl)
      n356 = Square(x=w741) -> (x^2=w735:dbl)
      n357 = Power Of X(1:w605, 2:3) -> (0:w598:dbl)
      n358 = Power Of X(1:w544, 2:3) -> (0:w537:dbl)
      n359 = Power Of X(1:w680, 2:3) -> (0:w673:dbl)
      n360 = Power Of X(1:w741, 2:3) -> (0:w734:dbl)
      n361 = Multiply(x=1.36603, y=w605) -> (x*y=w620:dbl)
      n362 = Multiply(x=1.36603, y=w544) -> (x*y=w559:dbl)
      n363 = Multiply(x=1.36603, y=w680) -> (x*y=w695:dbl)
      n364 = Multiply(x=1.36603, y=w741) -> (x*y=w756:dbl)
      n365 = Multiply(x=w598, y=0.11116) -> (x*y=w597:dbl)
      n366 = Multiply(x=w599, y=-0.47719) -> (x*y=w596:dbl)
      n367 = Multiply(x=w537, y=0.11116) -> (x*y=w536:dbl)
      n368 = Multiply(x=w538, y=-0.47719) -> (x*y=w535:dbl)
      n369 = Multiply(x=w673, y=0.11116) -> (x*y=w672:dbl)
      n370 = Multiply(x=w674, y=-0.47719) -> (x*y=w671:dbl)
      n371 = Multiply(x=w734, y=0.11116) -> (x*y=w733:dbl)
      n372 = Multiply(x=w735, y=-0.47719) -> (x*y=w732:dbl)
      n373 = Compound Arithmetic op=unknown(w597, w596, w620) -> (w572:dbl)
      n374 = Compound Arithmetic op=unknown(w536, w535, w559) -> (w512:dbl)
      n375 = Compound Arithmetic op=unknown(w672, w671, w695) -> (w648:dbl)
      n376 = Compound Arithmetic op=unknown(w733, w732, w756) -> (w708:dbl)
      n377 = Subtract(x=w566, y=w572) -> (x-y=w569:dbl)
      n378 = Multiply(x=w572, y=w574) -> (x*y=w573:dbl)
      n379 = Subtract(x=w506, y=w512) -> (x-y=w509:dbl)
      n380 = Multiply(x=w512, y=w501) -> (x*y=w513:dbl)
      n381 = Subtract(x=w642, y=w648) -> (x-y=w645:dbl)
      n382 = Multiply(x=w648, y=w637) -> (x*y=w649:dbl)
      n383 = Subtract(x=w702, y=w708) -> (x-y=w705:dbl)
      n384 = Multiply(x=w708, y=w710) -> (x*y=w709:dbl)
      n385 = Multiply(x=w578, y=w569) -> (x*y=w570:dbl)
      n386 = Multiply(x=w517, y=w509) -> (x*y=w510:dbl)
      n387 = Multiply(x=w653, y=w645) -> (x*y=w646:dbl)
      n388 = Multiply(x=w714, y=w705) -> (x*y=w706:dbl)
      n389 = Add(x=w570, y=w573) -> (x+y=w565:dbl)
      n390 = Add(x=w510, y=w513) -> (x+y=w505:dbl)
      n391 = Add(x=w646, y=w649) -> (x+y=w641:dbl)
      n392 = Add(x=w706, y=w709) -> (x+y=w701:dbl)
      n393 = Multiply(x=w565, y=w485) -> (x*y=w564:dbl)
      n394 = Multiply(x=w505, y=w485) -> (x*y=w504:dbl)
      n395 = Multiply(x=w641, y=w629) -> (x*y=w640:dbl)
      n396 = Multiply(x=w701, y=w629) -> (x*y=w700:dbl)
      n397 = Subtract(x=w566, y=w564) -> (x-y=w498:dbl)
      n398 = Subtract(x=w506, y=w504) -> (x-y=w497:dbl)
      n399 = Subtract(x=w642, y=w640) -> (x-y=w632:dbl)
      n400 = Subtract(x=w702, y=w700) -> (x-y=w633:dbl)
      n401 = case shown="False" w500 {
        tunnel: [w777 w783] -> w484
        tunnel: w485 -> [_ w784]
        tunnel: w499 -> [w780 _]
        tunnel: w498 -> [w779 _]
        tunnel: w497 -> [w778 _]
        frame False {
          n402 = case shown="False" w780 {
            tunnel: [w781 w782] -> w777
            tunnel: w779 -> [_ w782]
            tunnel: w778 -> [w781 _]
            frame False {
            }
            frame True {
            }
          }
        }
        frame True {
          n403 = Subtract(x=1.0, y=w784) -> (x-y=w783:dbl)
        }
      }
      n404 = case shown="False" w636 {
        tunnel: [w786 w792] -> w635
        tunnel: w629 -> [_ w793]
        tunnel: w634 -> [w789 _]
        tunnel: w633 -> [w788 _]
        tunnel: w632 -> [w787 _]
        frame False {
          n405 = case shown="False" w789 {
            tunnel: [w790 w791] -> w786
            tunnel: w788 -> [_ w791]
            tunnel: w787 -> [w790 _]
            frame False {
            }
            frame True {
            }
          }
        }
        frame True {
          n406 = Subtract(x=1.0, y=w793) -> (x-y=w792:dbl)
        }
      }
      n407 = Multiply(x=w484, y=w466) -> (x*y=w467:dbl)
      n408 = Multiply(x=w635, y=w477) -> (x*y=w476:dbl)
      n409 = case shown="False" w470 {
        tunnel: 0.0 -> [w762 w769]
        tunnel: w477 -> [w761 w776]
        tunnel: w476 -> [w760 w775]
        tunnel: "AFP Efficiency" -> [_ w763]
        tunnel: [w760 w771] -> w474
        tunnel: [w761 w770] -> w473
        tunnel: [w762 w769] -> w472
        tunnel: w467 -> [w759 w768]
        tunnel: [w759 w767] -> w468
        tunnel: w466 -> [w758 w766]
        tunnel: [w758 w764] -> w465
        frame False {
        }
        frame True {
          n410 = Negate(x=w766) -> (-x=w765:dbl)
          n411 = Negate(x=w768) -> (-x=w774:dbl)
          n412 = Negate(x=w775) -> (-x=w773:dbl)
          n413 = Negate(x=w776) -> (-x=w772:dbl)
          n414 = Multiply(x=w765, y=w763) -> (x*y=w764:dbl)
          n415 = Multiply(x=w774, y=w763) -> (x*y=w767:dbl)
          n416 = Multiply(x=w773, y=w763) -> (x*y=w771:dbl)
          n417 = Multiply(x=w772, y=w763) -> (x*y=w770:dbl)
        }
      }
    }
    n418 = Divide(x=12.0, y=500.0) -> (x/y=w71:dbl)
    n419 = Divide(x=12.0, y=500.0) -> (x/y=w109:dbl)
    n420 = Divide(x=12.0, y=500.0) -> (x/y=w113:dbl)
    n421 = Divide(x=12.0, y=500.0) -> (x/y=w67:dbl)
    n422 = Multiply(x=w63, y=w71) -> (x*y=→"upper R-value AFP":dbl)
    n423 = Multiply(x=w102, y=w109) -> (x*y=→"lower R-value":dbl)
    n424 = Multiply(x=w105, y=w113) -> (x*y=→"upper R-value":dbl)
    n425 = Multiply(x=w60, y=w67) -> (x*y=→"lower R-value AFP":dbl)
    n426 = case shown="True" w151 {
      tunnel: w155 -> [_ w454]
      tunnel: w54 -> [w450 w453]
      tunnel: w54 -> [_ w452]
      tunnel: [w450 w452] -> w154
      tunnel: [w449 w451] -> w142
      tunnel: w145 -> [w449 _]
      frame False {
      }
      frame True {
        n427 = Subtract(x=w454, y=w453) -> (x-y=w451:dbl[])
      }
    }
    n428 = case shown="True" w151 {
      tunnel: w169 -> [_ w460]
      tunnel: w160 -> [w456 w459]
      tunnel: w168 -> [_ w458]
      tunnel: [w456 w458] -> w152
      tunnel: [w455 w457] -> w141
      tunnel: w145 -> [w455 _]
      frame False {
      }
      frame True {
        n429 = Subtract(x=w460, y=w459) -> (x-y=w457:dbl[])
      }
    }
    n430 = Add(x=w154, y=w44) -> (x+y=w34:dbl[])
    n431 = Add(x=w142, y=w44) -> (x+y=w36:dbl[])
    n432 = Add(x=w45, y=w141) -> (x+y=w38:dbl[])
    n433 = Add(x=w45, y=w152) -> (x+y=w40:dbl[])
    n434 = call "FitAndSubtract.vi"("Array 4"=w31, "Array 3"=w32, "Numeric"=w33, "Array in"=w34) -> ("Array out"=w35:dbl[])  [unwired: 6 in, 1 out]
    n435 = call "FitAndSubtract.vi"("Array 4"=w31, "Array 3"=w32, "Numeric"=w33, "Array in"=w36) -> ("Array out"=w37:dbl[])  [unwired: 6 in, 1 out]
    n436 = call "FitAndSubtract.vi"("Array 4"=w31, "Array 3"=w32, "Numeric"=w33, "Array in"=w38) -> ("Array out"=w41:dbl[])  [unwired: 6 in, 1 out]
    n437 = Bundle(w32, w40) -> (w194:cluster{dbl[], dbl[]})  [unwired: 1 in]
    n438 = call "FitAndSubtract.vi"("Array 4"=w31, "Array 3"=w32, "Numeric"=w33, "Array in"=w40) -> ("Best Polynomial Fit"=w39:dbl[], "Array out"=w42:dbl[])  [unwired: 6 in]
    n439 = Bundle(w32, "Best Polynomial Fit"=w39) -> (w128:cluster{dbl[], "Best Polynomial Fit":dbl[]})  [unwired: 1 in]
    n440 = call "rhozero.vi"("Array in"=w35) -> ("Array out"=w149:dbl[])  [unwired: 10 in]
    n441 = call "rhominus.vi"("Array"=w42, "Array 2"=w35) -> ("Array 3"=w148:dbl[])  [unwired: 9 in]
    n442 = Add(x=w41, y=w37) -> (x+y=w143:dbl[])
    n443 = Subtract(x=w41, y=w37) -> (x-y=w144:dbl[])
    n444 = call "rhoplus.vi"("Array 3"=w35, "Array in"=w42) -> ("Array out"=w150:dbl[])  [unwired: 9 in]
    n445 = Build Array(w194, w128) -> (→"Signal and Fit (P)":cluster{dbl[], "Best Polynomial Fit":dbl[]}[])
    n446 = Divide(x=w143, y=w140) -> (x/y=w139:dbl[])
    n447 = Subtract(x=w150, y=w149) -> (x-y=w137:dbl[])
    n448 = Divide(x=w144, y=w140) -> (x/y=w138:dbl[])
    n449 = Bundle(w32, "Array out"=w149) -> (→"Rho_0":cluster{dbl[], "Array out":dbl[]})  [unwired: 1 in]
    n450 = Bundle(w32, "Array out"=w150) -> (→"Rho_+":cluster{dbl[], "Array out":dbl[]})  [unwired: 1 in]
    n451 = Subtract(x=w149, y=w148) -> (x-y=w136:dbl[])
    n452 = Bundle(w32, "Array 3"=w148) -> (→"Rho_-":cluster{dbl[], "Array 3":dbl[]})  [unwired: 1 in]
    n453 = Reverse 1D Array(array=w139) -> (reversed array=w147:dbl[])
    n454 = Reverse 1D Array(array=w138) -> (reversed array=w146:dbl[])
    n455 = Divide(x=w147, y=w140) -> (x/y=w48:dbl[])
    n456 = Divide(x=w146, y=w140) -> (x/y=w49:dbl[])
    n457 = Add(x=w136, y=w48) -> (x+y=w134:dbl[])
    n458 = Add(x=w137, y=w49) -> (x+y=w135:dbl[])
    n459 = Subtract(x=w135, y=w134) -> (x-y=w122:dbl[])
    n460 = Add(x=w134, y=w135) -> (x+y=w19:dbl[])
    n461 = Bundle(w32, w135) -> (w129:cluster{dbl[], dbl[]})  [unwired: 1 in]
    n462 = Bundle(w32, w134) -> (w130:cluster{dbl[], dbl[]})  [unwired: 1 in]
    n463 = Add Array Elements(numeric array=w19) -> (sum=w124:dbl)
    n464 = Add Array Elements(numeric array=w122) -> (sum=w123:dbl)
    n465 = Bundle(w32, w122) -> (→"Corrected Data (Q)":cluster{dbl[], dbl[]})  [unwired: 1 in]
    n466 = Bundle(w32, w19) -> (w131:cluster{dbl[], dbl[]})  [unwired: 1 in]
    n467 = Array To Spreadsheet String(delimiter (Tab)=",", array=w19, 3:"%f") -> (spreadsheet string=w30:string)
    n468 = Format Into String(format string="%d", initial string="", w16) -> (resulting string=w84:string)  [unwired: 1 in, 1 out]
    n469 = Build Array(w131, w129, w130) -> (→"Corrected Data (P)":cluster{dbl[], dbl[]}[])
    n470 = Number To Fractional String(number="Saturation\nPolarization", precision (6)=i16 2) -> (F-format string=w28:string)  [unwired: 2 in]
    n471 = Divide(x=12.0, y=500.0) -> (x/y=w120:dbl)
    n472 = Divide(x=12.0, y=500.0) -> (x/y=w114:dbl)
    n473 = Multiply(x=w124, y=w120) -> (x*y=w121:dbl)
    n474 = Multiply(x=w123, y=w114) -> (x*y=w117:dbl)
    n475 = Absolute Value(x=w121) -> (abs(x)=w74:dbl)
    "Reimann\nsum of P" <- w74
    n476 = Concatenate Strings(w84, ",", w28, ",", w30) -> (w81:string)
    n477 = Absolute Value(x=w117) -> (abs(x)=w101:dbl)
    "Reimann \nsum of Q" <- w101
    n478 = Write to Text File(file (use dialog)=w90, text=w81, error in=w89) -> (refnum out=w88:refnum<file>, error out=w87:errorcluster)  [unwired: 1 in, 1 out]
    n479 = Square(x=w74) -> (x^2=w72:dbl)
    n480 = Bundle(w74, w101) -> (→"Total Polarization (P)":cluster{dbl, dbl})  [unwired: 1 in]
    n481 = Multiply(x=3, y=w72) -> (x*y=w76:dbl)
    n482 = call "Ann_int.vi"("Optimizer"="Optimizer", "Adam Data In"=w18, "Loss Function"="Loss Function", "Target"="Saturation\nPolarization", "Parameters"=w24, "Training?"="Training?", "Data"=w19) -> ("Adjusted Parameters"=w25:T3, "Error"=→"NN Error" →"NN Testing Error":dbl, "Output"=→"NN Output":dbl, "Adam Data Out"=w17:T1)  [unwired: 1 in]
    n483 = Subtract(x=4, y=w76) -> (x-y=w73:dbl)
    n484 = Square Root(x=w73) -> (sqrt(x)=w78:dbl)
    n485 = Subtract(x=2, y=w78) -> ()  [unwired: 1 out]
  }
  n486 = invoke class="VI" method="Default Vals.Reinit All"(reference=w14) -> ()  [unwired: 2 in, 3 out]
  n487 = property on="Total Polarization (P)" class="WFChart (strict)"("History Data"=cluster{dbl, dbl}[] []) -> ()  [unwired: 2 in, 2 out]
  n488 = property on="NN Testing Error" class="WFChart (strict)"("History Data"=dbl[] []) -> ()  [unwired: 2 in, 2 out]
  n489 = Close File(refnum=w10, error in=w9) -> ()  [unwired: 2 out]
  n490 = Flatten To XML(anything=w5) -> (xml string=w4:string)
  n491 = call-poly <vilib>:"Write to XML File.vi"("XML Input"=w4, "XML File Path"="Parameters File Path") -> ()  [unwired: 7 in, 3 out]
